vi "DAQ.GetPrivateEvents.vi"(8 "error in (no error)":errorcluster, 11 "Instrument.DAQ":refnum<class "Instrument.DAQ.lvclass">) -> (0 "error out":errorcluster, 2 "DAQ Private Events":T1, 3 "Instrument.DAQ":refnum<class "Instrument.DAQ.lvclass">)   [LabVIEW 2019, in "Instrument.Lockin.lvlib" / "Instrument.DAQ.lvclass"]
doc: "---------------------------------------------------------------\nJKI State Machine Objects™\nhttp://jki.net/state-machine-objects/\nCopyright (C) 2005-2015, JKI <info@jki.net>\nALL RIGHTS RESERVEDJKI State Machine Objects (SMO) 1.0.0.4\nJKI - JKI\nCopyright (c) 2015, JKI"
uses:
  Instrument.DAQ.lvclass
  Typedefs/PrivateEvents--Cluster.ctl
  Typedefs/PrivateEvents--DAQ.setAOconfig.ctl
  Typedefs/DAQ.Config.AO--Cluster--Array.ctl
  Typedefs/DAQ.Config.AO.Range--enum.ctl
  Typedefs/DAQ.TerminalConfiguration--ring.ctl
  Typedefs/DAQ.Type--enum.ctl
  Typedefs/PrivateEvents--DAQ.setAIconfig.ctl
  Typedefs/DAQ.Config.AI--Cluster--Array.ctl
  Typedefs/DAQ.Config.AI.Coupling--enum.ctl
  Typedefs/DAQ.Config.AI.Range--enum.ctl
  DAQmx/typedefs/Simulation Mode--enum.ctl
  Typedefs/PrivateEvents--DAQ.setAO.ctl
  Typedefs/AO.Channel--Cluster--Array.ctl
  Typedefs/AO.Channel--Cluster.ctl
  Typedefs/AO.Channel.Function--Enum.ctl
  Typedefs/PrivateEvents--DAQ.setREF.ctl
  Typedefs/REF.Channel--Cluster--Array.ctl
  Typedefs/REF.Channel--Cluster.ctl
  Typedefs/PrivateEvents--DAQ.setSampling.ctl
  Typedefs/DAQ.Sampling--Cluster.ctl
  Typedefs/DAQ.Sampling.Sampling--Cluster.ctl
  Typedefs/PrivateEvents--DAQ.setState.ctl
  Typedefs/State--enum.ctl
  Typedefs/PrivateEvents--DAQ.setInputGain.ctl
  Typedefs/PrivateEvents--DAQ.setSweep.ctl
  Typedefs/Sweep.Configuration--Cluster.ctl
  Typedefs/Sweep.Channel--Cluster--Array.ctl
  Typedefs/Sweep.Channel--Cluster.ctl
  Typedefs/Sweep.Pattern--Enum.ctl
  Typedefs/PrivateEvents--DAQ.measureOffset.ctl
  Typedefs/PrivateEvents--DAQ.zeroOffset.ctl
  Typedefs/PrivateEvents--DAQ.setPreFilter.ctl
  Typedefs/Configuration.Prefilter--Cluster.ctl
  Typedefs/PrivateEvents--DAQ.autoConfigureDAQ.ctl
  Typedefs/PrivateEvents--DAQ.setCalibration.ctl
  Typedefs/PrivateEvents--DAQ.setAI.ctl
  Typedefs/AI.Channel--Cluster--Array.ctl
  Typedefs/AI.Channel--Cluster.ctl
  Typedefs/PrivateEvents--DAQ.zeroPhase.ctl
  Typedefs/PrivateEvents--DAQ.setAmplitudeLimit.ctl
  Typedefs/Configuration.AmplitudeLimit--Cluster.ctl
  Typedefs/PrivateEvents--DAQ.setLinkFrequencies.ctl
  Typedefs/Configuration.LinkFrequencies--Cluster.ctl
  Typedefs/PrivateEvents--DAQ.showUI.ctl
  Typedefs/PrivateEvents--DAQ.setInputOffset.ctl
  Typedefs/PrivateEvents--DAQ.setDCLimit.ctl
  Typedefs/Configuration.DCLimit--Cluster.ctl
  Typedefs/PrivateEvents--DAQ.setDutyCycle.ctl
  Typedefs/Configuration.DutyCycle--Cluster.ctl
  Instrument.DAQ.lvclass/Instrument.DAQ.ctl
  DAQmx/DAQmx.lvclass
panel:
  # "For instructions on how to use the JKI State Machine Objects, examples and video tutorials, visit:\nhttp://jki.net/state-machine-objects/\n\nJKI State Machine Objects™\nhttp://jki.net/state-machine-objects/\nCopyright (C) 2005-2015, JKI <info@jki.net>\nALL RIGHTS RESERVED"
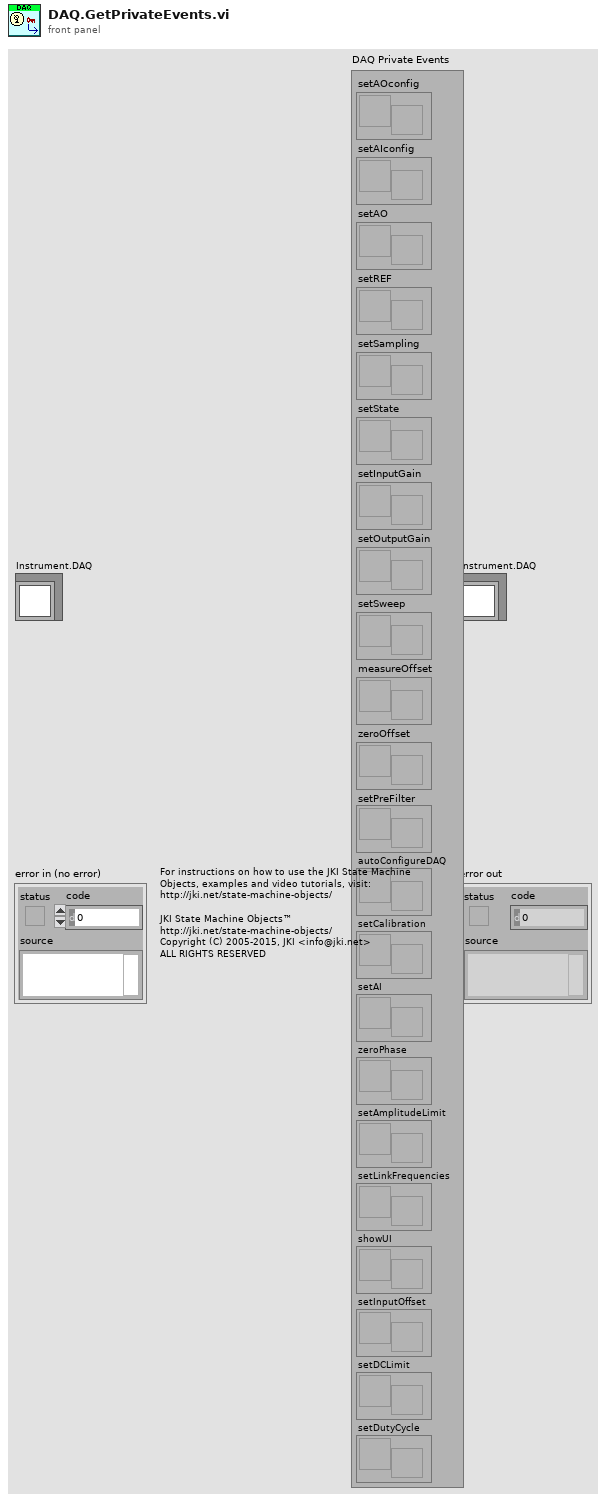
[diagram p1: front panel]
types:
  T1 = typedef "Instrument.Lockin.lvlib/Instrument.DAQ.lvclass/PrivateEvents--Cluster.ctl" = cluster{"setAOconfig":refnum<user-event>, "setAIconfig":refnum<user-event>, "setAO":refnum<user-event>, "setREF":refnum<user-event>, "setSampling":refnum<user-event>, "setState":refnum<user-event>, "setInputGain":refnum<user-event>, "setOutputGain":refnum<user-event>, "setSweep":refnum<user-event>, "measureOffset":refnum<user-event>, "zeroOffset":refnum<user-event>, "setPreFilter":refnum<user-event>, "autoConfigureDAQ":refnum<user-event>, "setCalibration":refnum<user-event>, "setAI":refnum<user-event>, "zeroPhase":refnum<user-event>, "setAmplitudeLimit":refnum<user-event>, "setLinkFrequencies":refnum<user-event>, "showUI":refnum<user-event>, "setInputOffset":refnum<user-event>, "setDCLimit":refnum<user-event>, "setDutyCycle":refnum<user-event>}
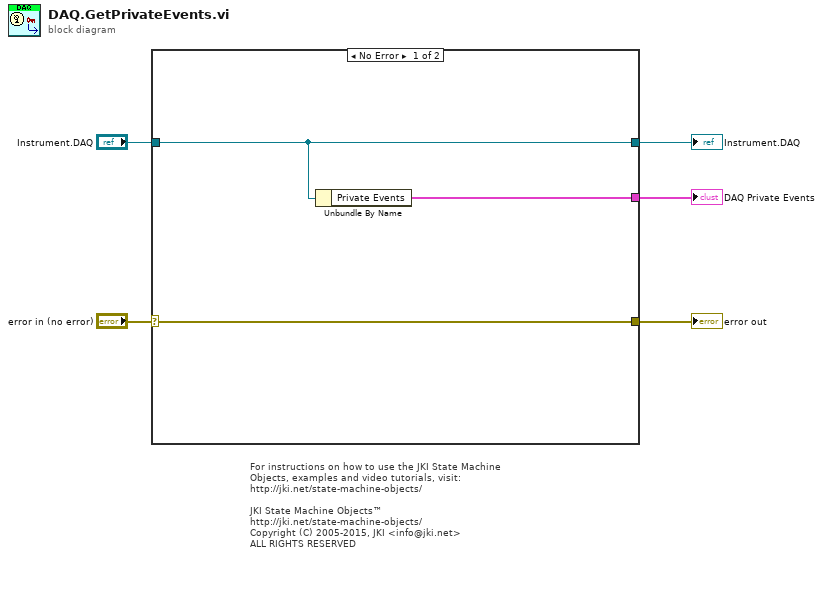
[diagram p0: block diagram]
diagram:
  # "For instructions on how to use the JKI State Machine Objects, examples and video tutorials, visit:\nhttp://jki.net/state-machine-objects/\n\nJKI State Machine Objects™\nhttp://jki.net/state-machine-objects/\nCopyright (C) 2005-2015, JKI <info@jki.net>\nALL RIGHTS RESERVED"
  n1 = case shown="No Error" "error in (no error)" {
    selector: "error in (no error)" -> [w7 w9]
    tunnel: "Instrument.DAQ" -> [w6 w10]
    tunnel: [w7 w9] -> w4
    tunnel: [w6 w10] -> w3
    tunnel: [w8 _] -> w1
    frame No Error {
      n2 = Unbundle By Name(w6) -> ("Private Events"=w8:T1)
    }
    frame Error {
    }
  }
  "error out" <- w4
  "Instrument.DAQ" <- w3
  "DAQ Private Events" <- w1
